vi "Modem Status Interpret Received CMD.vi"(8 "error in (no error)":errorcluster, 9 "Modem Status Raw Analog Data":T1, 10 "Msg Body":string, 11 "Address Table":u8[](array[numeric])) -> (0 "error out":errorcluster, 1 "Modem Status Raw Analog Data Out":T1)   [LabVIEW 2011]
uses:
  Modem Status Raw Analog Data Cluster.ctl
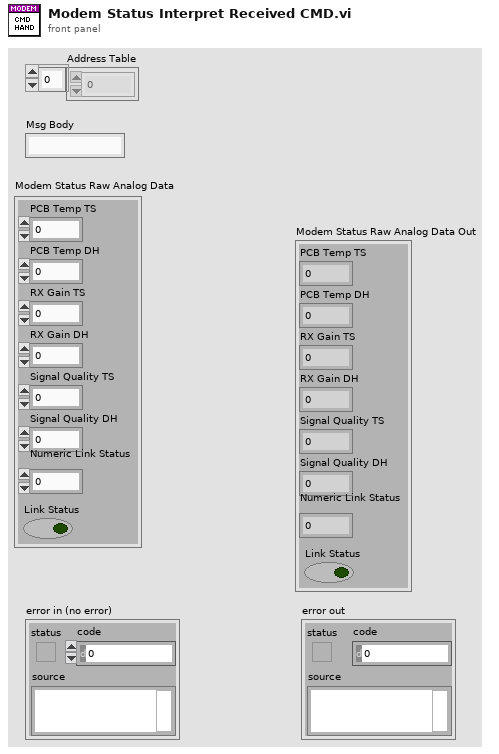
[diagram p1: front panel]
types:
  T1 = typedef "Modem Status Raw Analog Data Cluster.ctl" = cluster{"PCB Temp TS":dbl, "PCB Temp DH":dbl, "RX Gain TS":dbl, "RX Gain DH":dbl, "Signal Quality TS":dbl, "Signal Quality DH":dbl, "Numeric Link Status":dbl, "Link Status":bool}
  T2 = enum8{"LINK STATUS", "PCB TEMP TS", "PCB TEMP DH", "RX GAIN TS", "RX GAIN DH", "SIGNAL_QUALITY_DH", "SIGNAL_QUALITY_TS", "Unknown"}
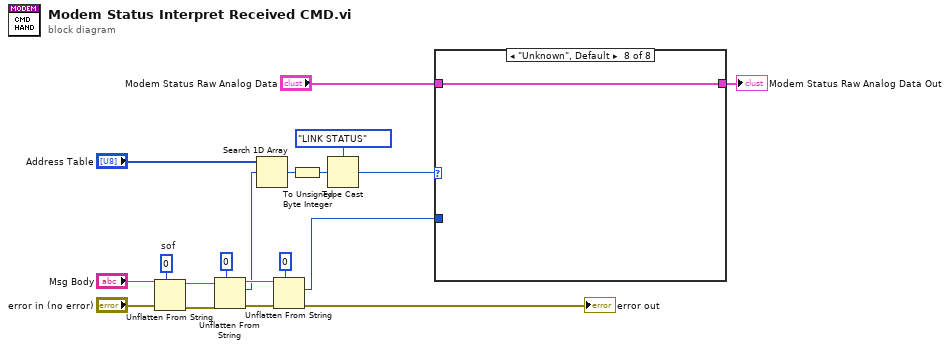
[diagram p0: block diagram]
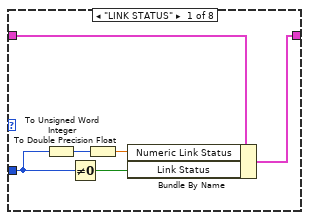
[diagram p2: hidden frame]
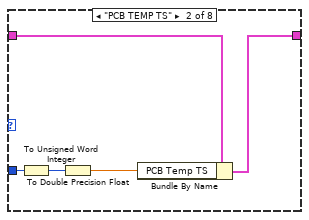
[diagram p3: hidden frame]
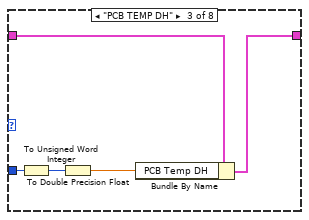
[diagram p4: hidden frame]
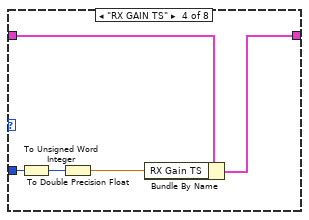
[diagram p5: hidden frame]
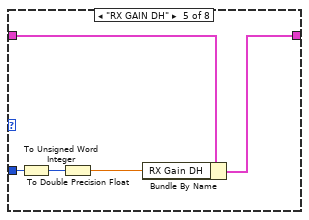
[diagram p6: hidden frame]
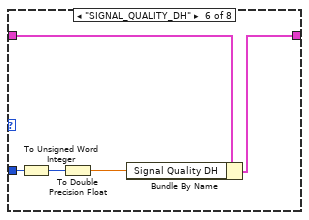
[diagram p7: hidden frame]
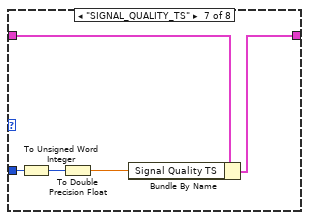
[diagram p8: hidden frame]
diagram:
  w5 = u8 0  # sof
  n1 = Unflatten From String(type=w5, binary string="Msg Body", error in (no error)="error in (no error)") -> (rest of the binary string=w1:string, error out=w2:errorcluster)  [unwired: 2 in, 1 out]
  n2 = Unflatten From String(type=u8 0, binary string=w1, error in (no error)=w2) -> (rest of the binary string=w17:string, value=w10:u8, error out=w15:errorcluster)  [unwired: 2 in]
  n3 = Search 1D Array(1D array="Address Table", element=w10) -> (index of element=w11:i32)  [unwired: 1 in]
  n4 = Unflatten From String(type=u32 0, binary string=w17, error in (no error)=w15) -> (value=w18:u32, error out=→"error out":errorcluster)  [unwired: 2 in, 1 out]
  n5 = To Unsigned Byte Integer(number=w11) -> (unsigned 8bit integer=w12:u8)
  n6 = Type Cast(type=T2."LINK STATUS", x=w12) -> (*(type *) &x=w14:T2)
  n7 = case shown="\"Unknown\", Default" w14 {
    tunnel: w18 -> [w22 w30 w35 w40 w45 w50 w55 _]
    tunnel: "Modem Status Raw Analog Data" -> [w24 w28 w33 w38 w43 w48 w53 w56]
    tunnel: [w23 w27 w32 w37 w42 w47 w52 w56] -> w6
    frame "LINK STATUS" {
      n8 = To Unsigned Word Integer(number=w22) -> (unsigned 16bit integer=w25:u16)
      n9 = Not Equal To 0?(x=w22) -> (x != 0?=w21:bool)
      n10 = To Double Precision Float(number=w25) -> (double precision float=w20:dbl)
      n11 = Bundle By Name(cluster=w24, "Numeric Link Status"=w20, "Link Status"=w21) -> (w23:T1)
    }
    frame "PCB TEMP TS" {
      n12 = To Unsigned Word Integer(number=w30) -> (unsigned 16bit integer=w29:u16)
      n13 = To Double Precision Float(number=w29) -> (double precision float=w26:dbl)
      n14 = Bundle By Name(cluster=w28, "PCB Temp TS"=w26) -> (w27:T1)
    }
    frame "PCB TEMP DH" {
      n15 = To Unsigned Word Integer(number=w35) -> (unsigned 16bit integer=w34:u16)
      n16 = To Double Precision Float(number=w34) -> (double precision float=w31:dbl)
      n17 = Bundle By Name(cluster=w33, "PCB Temp DH"=w31) -> (w32:T1)
    }
    frame "RX GAIN TS" {
      n18 = To Unsigned Word Integer(number=w40) -> (unsigned 16bit integer=w39:u16)
      n19 = To Double Precision Float(number=w39) -> (double precision float=w36:dbl)
      n20 = Bundle By Name(cluster=w38, "RX Gain TS"=w36) -> (w37:T1)
    }
    frame "RX GAIN DH" {
      n21 = To Unsigned Word Integer(number=w45) -> (unsigned 16bit integer=w44:u16)
      n22 = To Double Precision Float(number=w44) -> (double precision float=w41:dbl)
      n23 = Bundle By Name(cluster=w43, "RX Gain DH"=w41) -> (w42:T1)
    }
    frame "SIGNAL_QUALITY_DH" {
      n24 = To Unsigned Word Integer(number=w50) -> (unsigned 16bit integer=w49:u16)
      n25 = To Double Precision Float(number=w49) -> (double precision float=w46:dbl)
      n26 = Bundle By Name(cluster=w48, "Signal Quality DH"=w46) -> (w47:T1)
    }
    frame "SIGNAL_QUALITY_TS" {
      n27 = To Unsigned Word Integer(number=w55) -> (unsigned 16bit integer=w54:u16)
      n28 = To Double Precision Float(number=w54) -> (double precision float=w51:dbl)
      n29 = Bundle By Name(cluster=w53, "Signal Quality TS"=w51) -> (w52:T1)
    }
    frame "Unknown", Default {
    }
  }
  "Modem Status Raw Analog Data Out" <- w6
